vi "slow_control_2_02.vi"() -> ()   [LabVIEW 2018]
uses:
  <vilib>/DAQmx/read.llb/DAQmx Read (Analog 1D DBL NChan 1Samp).vi
  <vilib>/DAQmx/create/channels.llb/DAQmx Create Channel (AI-Voltage-Basic).vi
  <vilib>/DAQmx/miscellaneous.llb/DAQmx Fill In Error Info.vi
  <instrlib>/Lake Shore 335/Lake Shore 335.lvlib
  <instrlib>/CAEN PSM/CAEN PSM.lvlib
panel:
  out "Det.P input #":i32
  out "Flow input #":i32
  out "Coldhead":dbl
  out "Heater":dbl
  out "Cycle number":i32
  out "TOBA tester":dbl[][](array[numeric])
  in  "Cycles to execute":dbl=5.0 format="%#_13g"
  out "Moving average Det. P":dbl
  in  "N samples":i32=20
  in  "Allows tabs on \nfront panel":T1(tab)
  in  "Give name if \"Other\"":string[](array[string])
  in  "Specify input":T2(array[ring])=[enum."Detector", enum."Low", enum."High", enum."Flow", enum."None", enum."None", enum."None", enum."None"]
  in  "Multipliers":dbl[](array[numeric])=[0.2, 1.0, 1.0, 28.409091, 1.0, 1.0, 1.0, 1.0]
  in  "Offsets\nsubtracted":dbl[](array[numeric])=[0.002, 0.0, 0.0, 0.44376, 0.0, 0.0, 0.0, 0.0]
  in  "physical channels":tag[](array[tag])=["9207/ai0", "9207/ai1", "9207/ai2", "9207/ai3", "9207/ai4", "9207/ai5", "9207/ai6", "9207/ai7"]
  in  "Heater range":u16(ring) items=["Off", "Low (On)", "Medium", "High"]
  in  "Setpoint (°C)":dbl=-100.0 format="%.1f"
  in  "PID settings":cluster{"P":dbl, "I":dbl, "D":dbl}={"P"=50.0, "I"=20.0, "D"=120.0}
  in  "COM-port LakeShore":refnum<visa-resource-name>
  in  "ID Query":bool=TRUE
  in  "COM-port CAEN 1":refnum<visa-resource-name>
  in  "COM-port CAEN 2":refnum<visa-resource-name>
  out "Temp B":dbl
  out "Temp A":dbl
  out "LakeShore readings 2":dbl[](array[numeric])
  out "Converted NI9207 Readings":dbl[](array[numeric])
  in  "Run lakeshore?":bool
  out "Detector pressure":dbl
  in  "T 20":bool
  in  "T 19":bool
  in  "T 18":bool
  in  "T 17":bool
  in  "T 16":bool
  in  "T 15":bool
  in  "Detector P":bool
  in  "Overpressure threshold":dbl
  in  "Underpressure threshold":dbl
  out "Comm. status":bool
  in  "High Temp threshold":dbl format="%#_13g"
  in  "Low Temp threshold":dbl format="%#_13g"
  in  "Ignore Initialization Errors":bool=TRUE caption="Ignore init. errors?"
  out "LakeShore status":bool
  out "NI mod1 (P) status":bool
  out "CAEN 1 status":bool
  out "CAEN 2 status":bool
  out "Initialization status":bool
  out "Heater power (%)":cluster{timestamp[], dbl[]}[](graph)
  out "Flow (SLPM)":cluster{timestamp[], dbl[]}[](graph)
  out "Pressure":cluster{timestamp[], dbl[]}[](graph)
  out "Phase Diagram":cluster{"X":dbl, "Y":dbl}[](graph)
  in  "Temp. Channel selector":string(combo)="Average 15 to 20"
  out "Temperature":cluster{timestamp[], dbl[]}[](graph)
  in  "N samples":i32=30
  out "Average Flow (SLPM)":dbl caption="Average Flow (SLPM), of"
  in  "Pause?":bool
  out "Integrated Flow (SL)":dbl
  in  "Reset?":bool
  out "LakeShore readings":dbl[](array[numeric])
  out "Temp. 1":dbl
  out "Temp. 2":dbl
  out "Temp. 3":dbl
  out "Temp. 4":dbl
  out "Temp. 5":dbl
  out "Temp. 6":dbl
  out "Temp. 7":dbl
  out "Temp. 8":dbl
  out "Temp. 9":dbl
  out "Temp. 10":dbl
  out "Temp. 11":dbl
  out "Temp. 12":dbl
  out "Temp. 13":dbl
  out "Temp. 14":dbl
  out "Temp. 15":dbl
  out "Temp. 16":dbl
  out "Temp. 17":dbl
  out "Temp. 18":dbl
  out "Temp. 19":dbl
  out "Temp. 20":dbl
  out "1 to 4":dbl[](array[numeric])
  out "5 to 8":dbl[](array[numeric])
  out "9 to 12":dbl[](array[numeric])
  out "13 to 16":dbl[](array[numeric])
  out "17 to 20":dbl[](array[numeric])
  in  "Temperature Channel selector":string(combo)="Average 15 to 20"
  out "Historical Large Phase Diagram":cluster{dbl[], dbl[]}[](graph)
  out "Large Phase Diagram":cluster{"X":dbl, "Y":dbl}[](graph)
  in  "Temperature Channel selector":string(combo)="Average 15 to 20"
  in  "Set to zero":bool
  out "Bottom gate":dbl(knob) scale=0.0..-3000.0
  out "Top gate":dbl(knob) scale=0.0..3000.0
  in  "Apply Voltage":bool
  in  "VSet (V)":dbl[](array[numeric])
  in  "IMax (uA)":dbl[](array[numeric])
  in  "VMax (V)":dbl[](array[numeric])
  out "Cathode":dbl(knob) scale=0.0..-5000.0
  out "Anode":dbl(knob) scale=0.0..4000.0
  out "PMT 2":dbl(knob) scale=0.0..1000.0
  out "PMT 1":dbl(knob) scale=1.0..1000.0
  out "Vmon (V)":dbl[](array[numeric])
  out "IMon (uA)":dbl[](array[numeric])
  in  "Read V every N cycles":i16=120
  in  "Reset anode":bool
  in  "Kill every Y minutes":i32=10
  in  "Keep off for X seconds":i32=10
  out "?":bool
  out "Killed":bool
  out "Restarted":bool
  out "Anode times":dbl[](array[numeric]) format="%_12f"
  out "Anode times 2":timestamp[](array[timestamp])
  in  "Kill voltage":bool
  in  "stop":bool
  out "Voltages":dbl[](array[numeric])
  out "Started up?":bool
  out "TOBA appended":dbl[][](array[numeric])
  in  "Read T every N cycles":i32=2
  out "Time until next cycle":dbl format="%.3g"
  in  "Time per cycle (s)":i32=2 caption="Time Target (s)"
  # "<- Proof of concept for New/Old T + New P"
  # "PMT 1"
  # "PMT 2"
  # "Anode"
  # "Cathode"
  # "Top gate"
  # "Bottom gate"
  # "Connection settings"
  # "Lakeshore settings"
  # "NI 9207 Voltage settings"
  # "Gain (P) (XX.X)"
  # "Reset (I) (XX.X)"
  # "Rate (D) (X.X%)"
  # "Move to Quick Temp tab ^"
  # "Alarm indicators"
  # "Thresholds"
  # "Alarm conditions"
  # "CAEN 1"
  # "Data"
  # "PMT 1"
  # "PMT 1"
  # "PMT 2"
  # "PMT 2"
  # "Anode"
  # "Anode"
  # "Cathode"
  # "Cathode"
  # "Top gate"
  # "Top gate"
  # "Bottom gate"
  # "Bottom gate"
  # "Settings"
  # "PMT 1"
  # "PMT 1"
  # "PMT 2"
  # "PMT 2"
  # "Anode"
  # "Anode"
  # "Cathode"
  # "Cathode"
  # "Top gate"
  # "Top gate"
  # "Bottom gate"
  # "Bottom gate"
  # "CAEN 2"
  # "PMT 1"
  # "PMT 2"
  # "Anode"
  # "Cathode"
  # "Needle gauges or other displays go here"
  # "Top gate"
  # "Bottom gate"
  # "Time of last reset"
  # "Time of last reactivation"
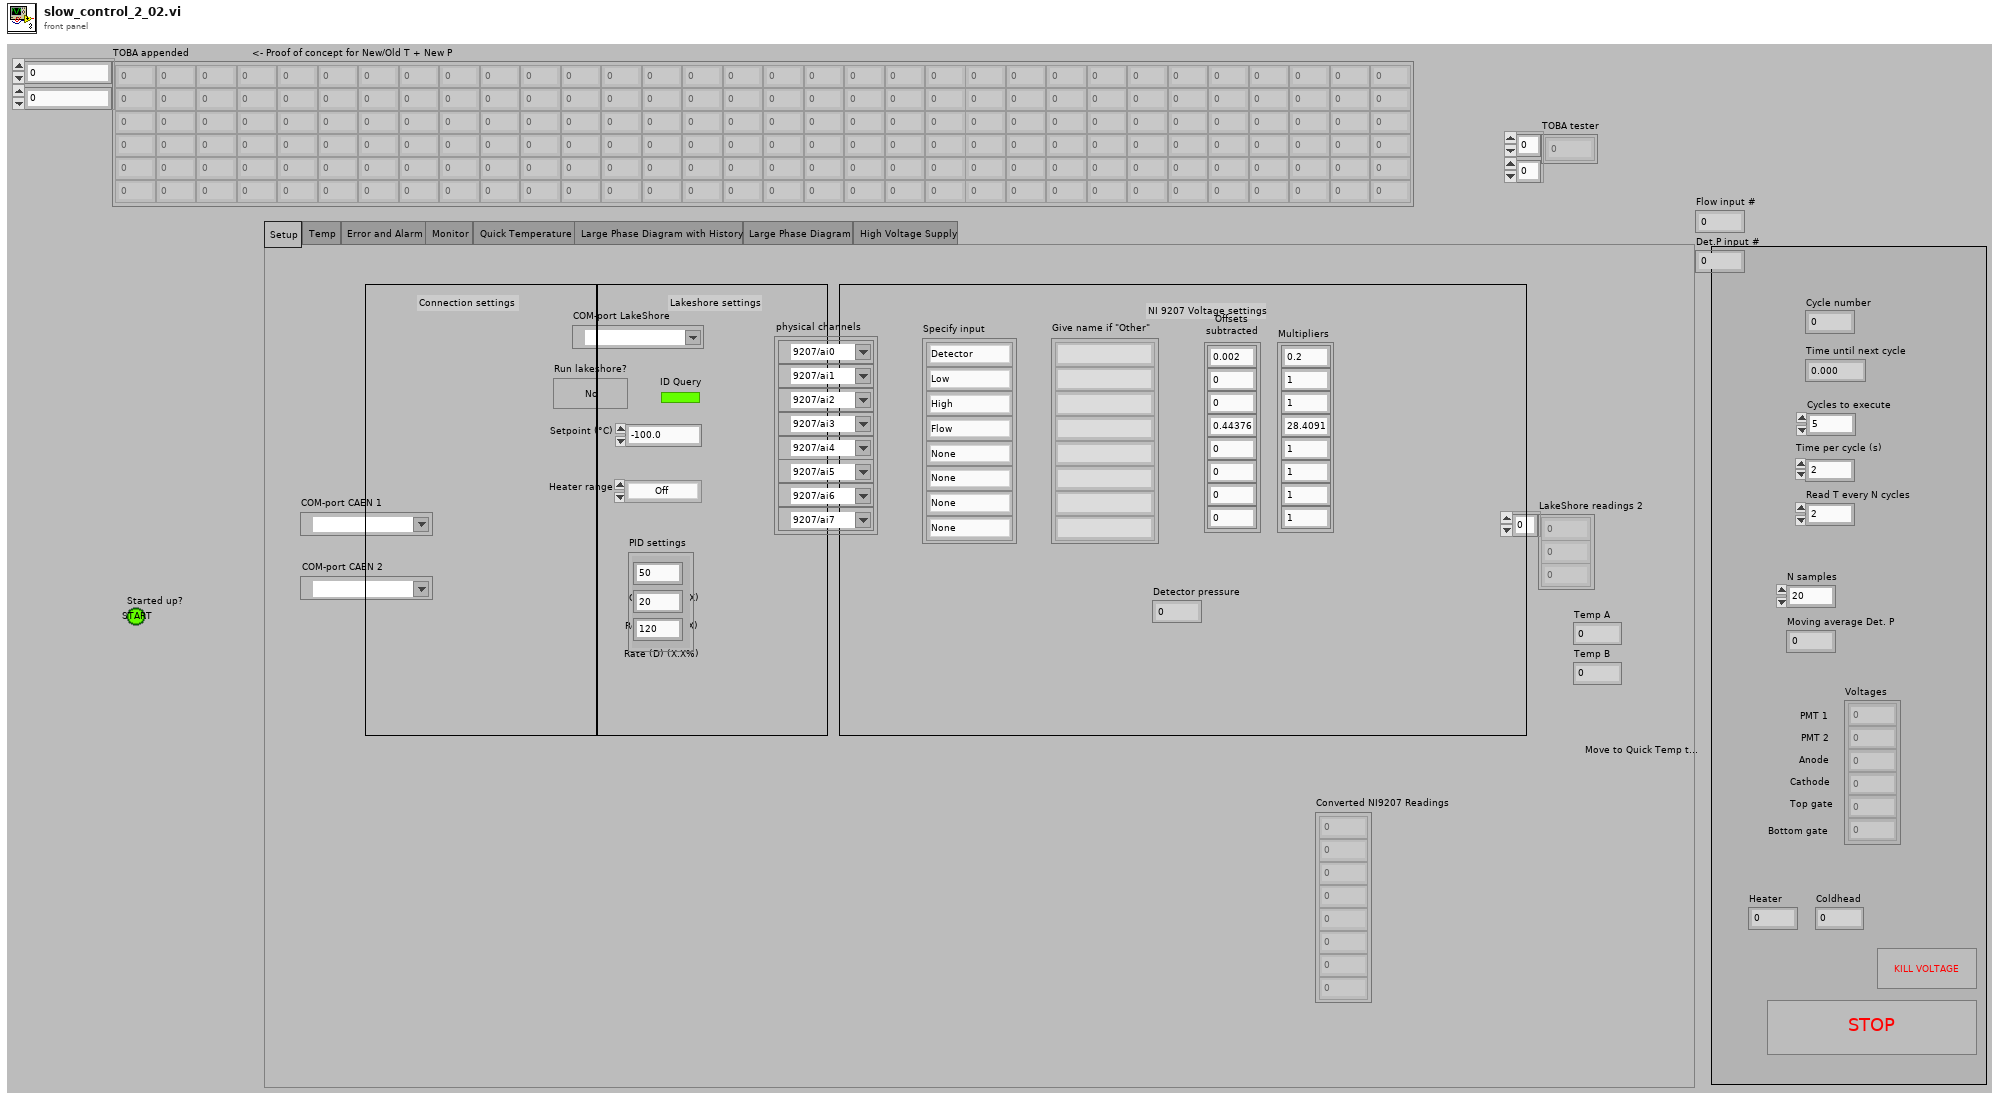
[diagram p1: front panel]
types:
  T1 = enum32{"Setup", "Temp", "Error and Alarm", "Monitor", "Quick Temperature", "Large Phase Diagram with History", "Large Phase Diagram", "High Voltage Supply"}
  T2 = enum16{"Detector", "Low", "High", "Flow", "Other", "None"}[]
  T3 = enum16{"Detector", "Low", "High", "Flow", "Other", "None"}
  T4 = cluster{"Baud Rate":u32, "Parity":u16, "Data Bits":u16, "Stop Bits":u16, "Flow Control":u16}
  T5 = cluster{"VISA resource name out":refnum<visa-resource-name>, "error out":errorcluster}
  T6 = cluster{"task out":refnum<k21>, "error out":errorcluster}
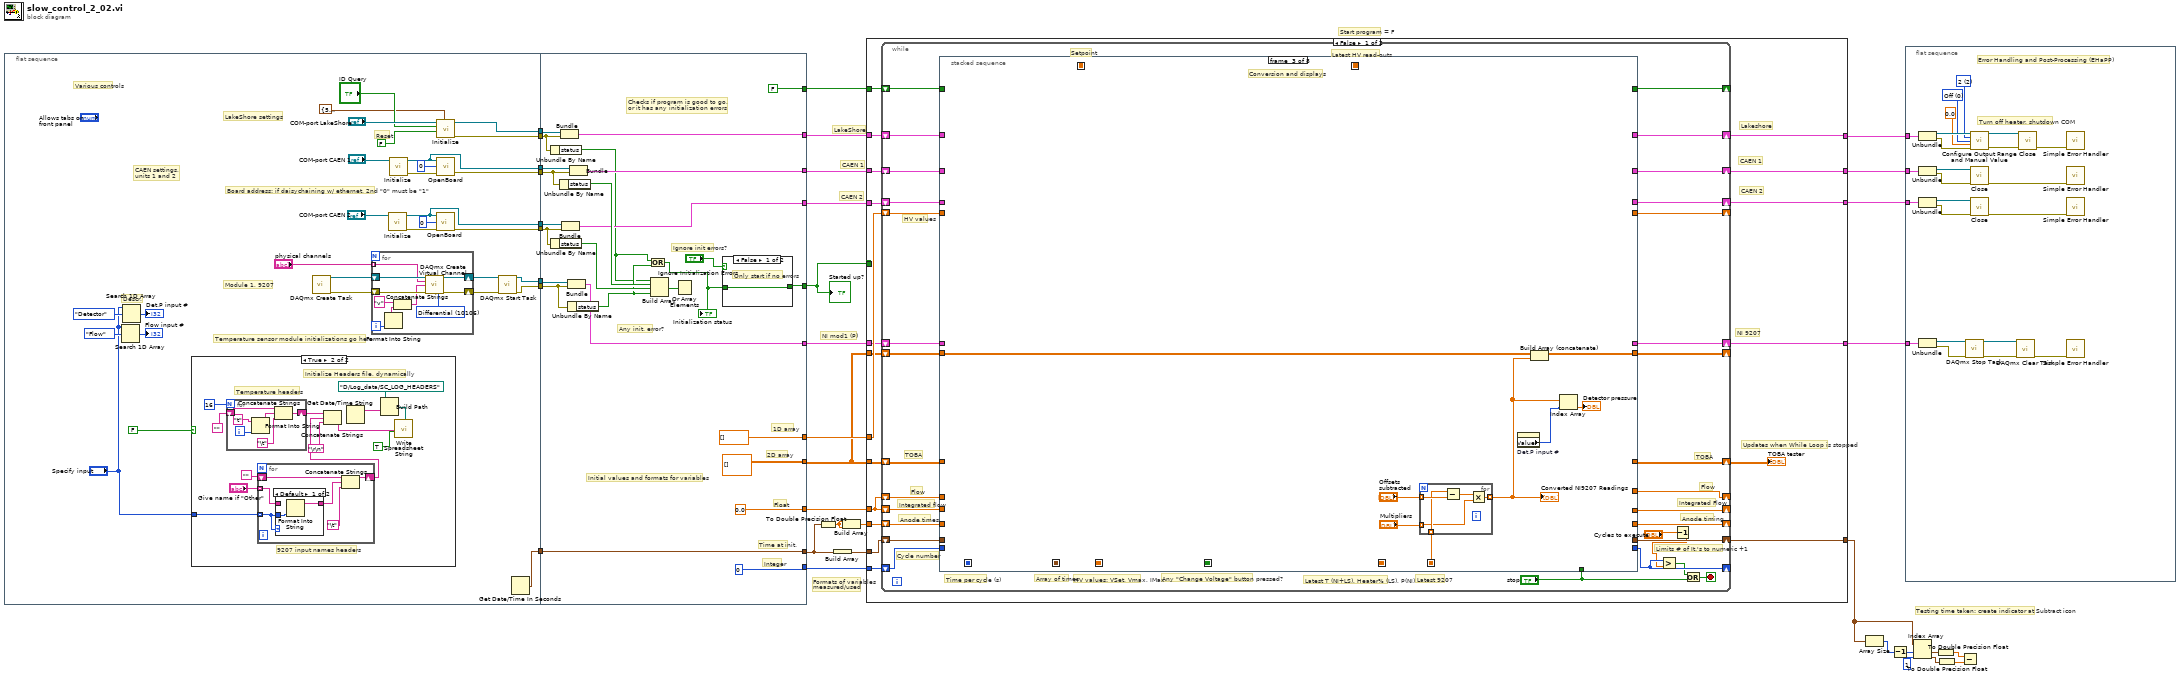
[diagram p0: block diagram]
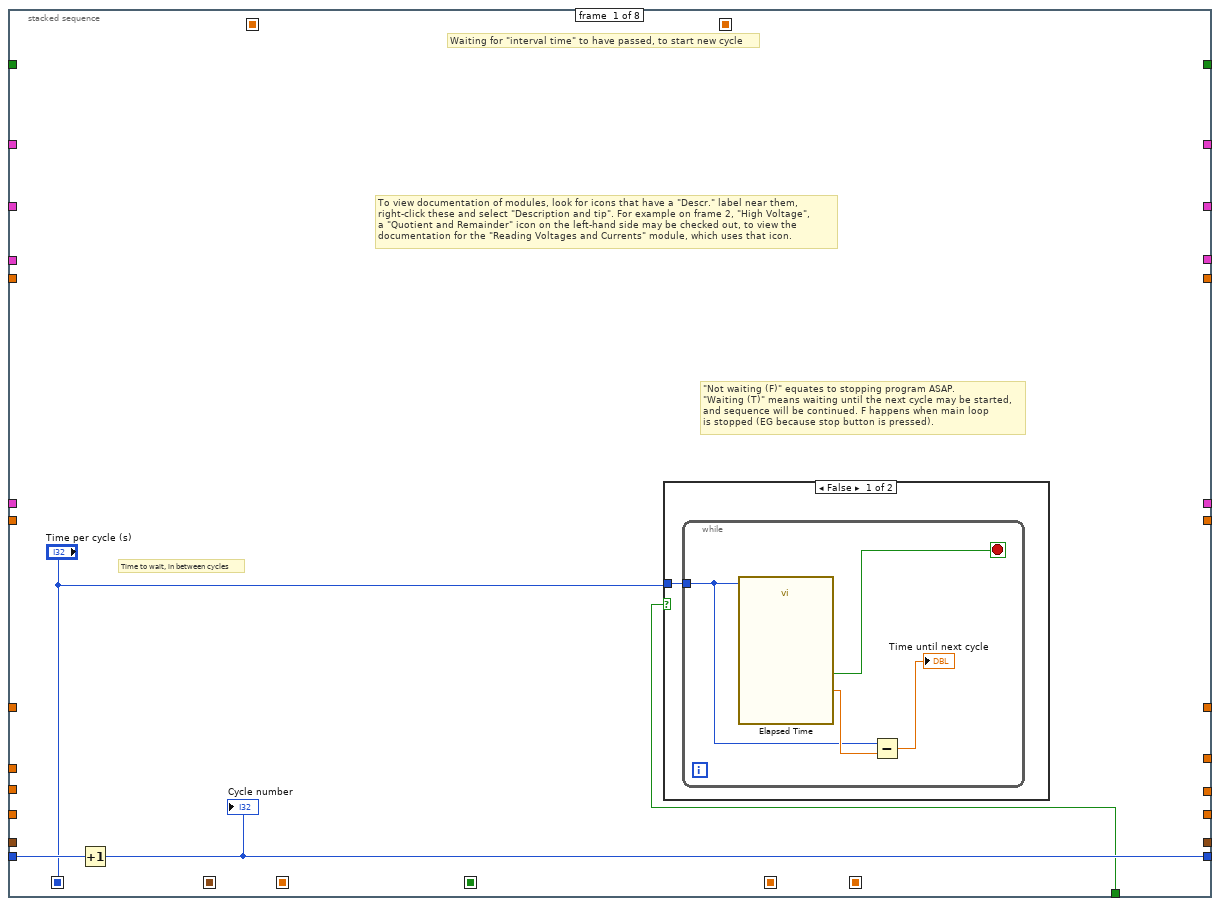
[diagram p2: hidden frame]
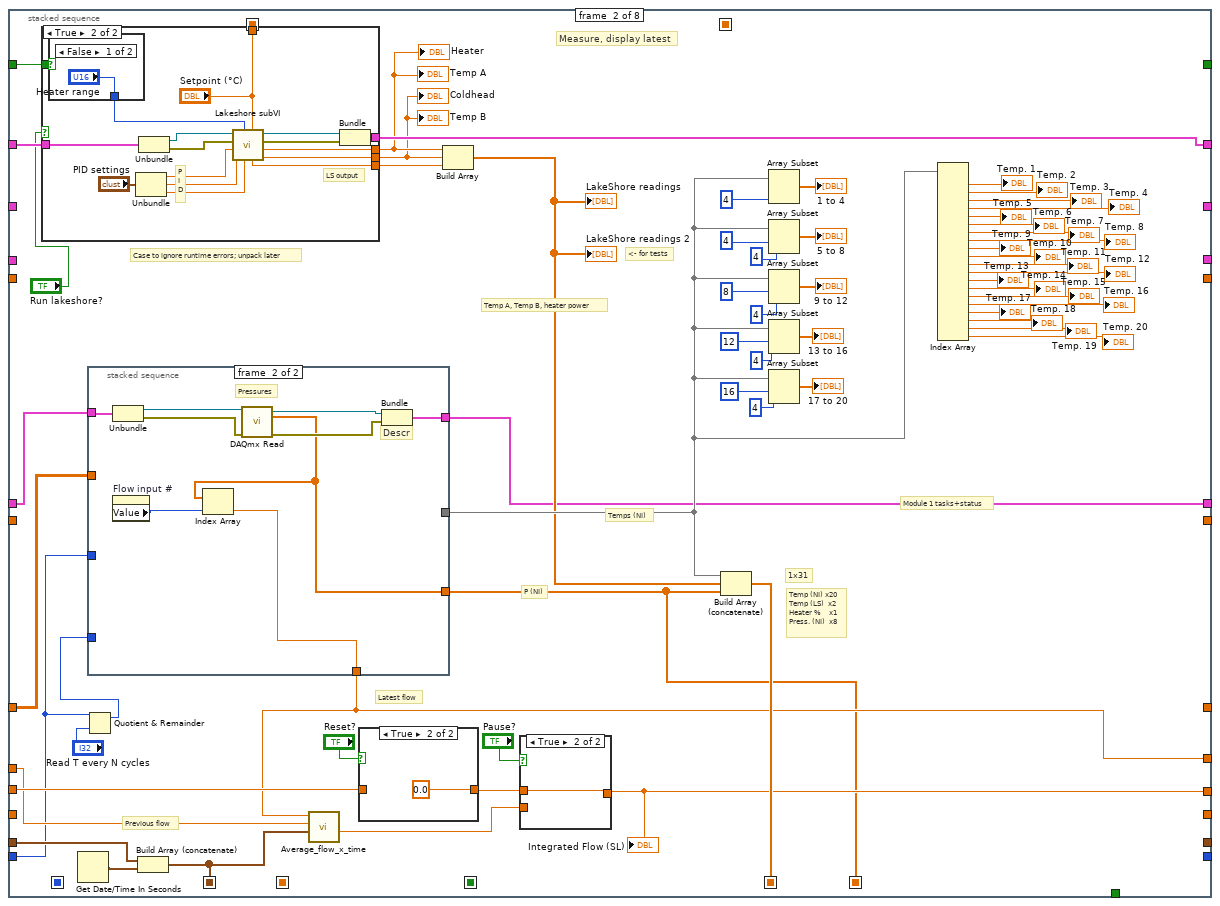
[diagram p4: hidden frame]
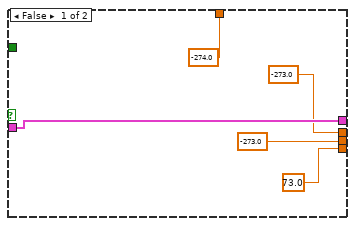
[diagram p5: hidden frame]
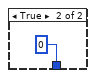
[diagram p6: hidden frame]
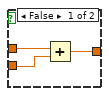
[diagram p8: hidden frame]
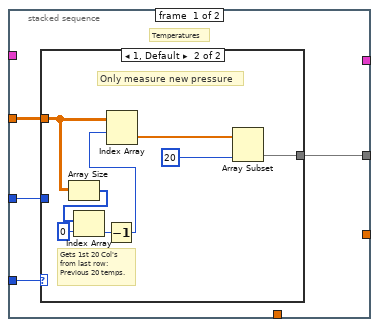
[diagram p9: hidden frame]
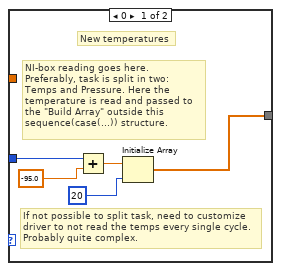
[diagram p10: hidden frame]
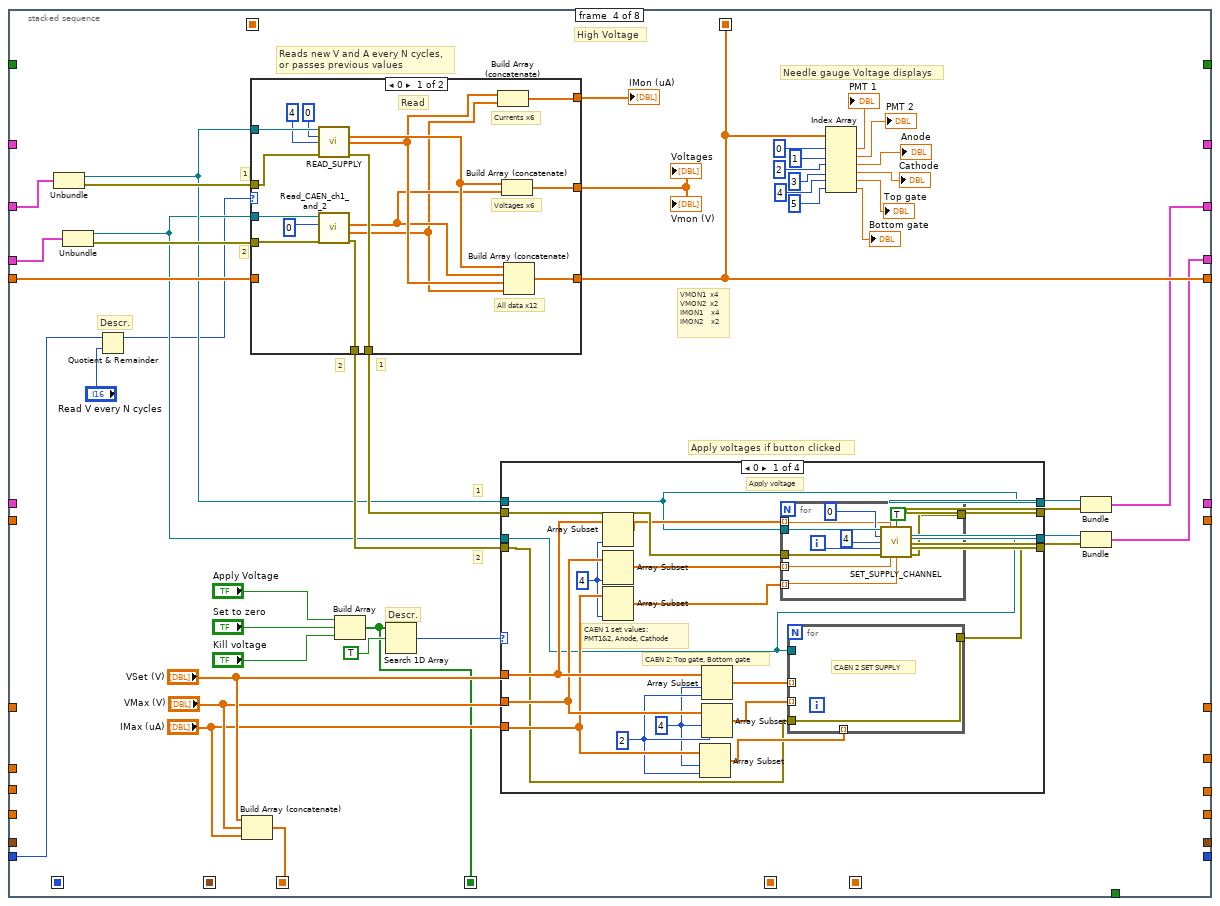
[diagram p11: hidden frame]
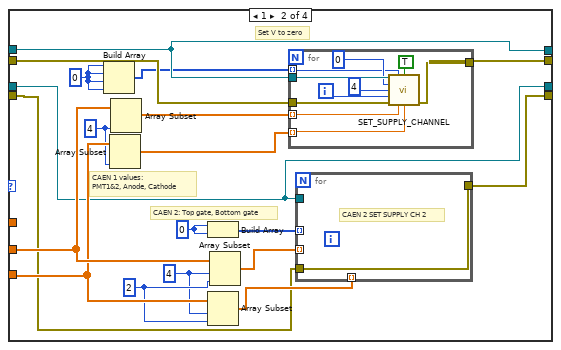
[diagram p12: hidden frame]
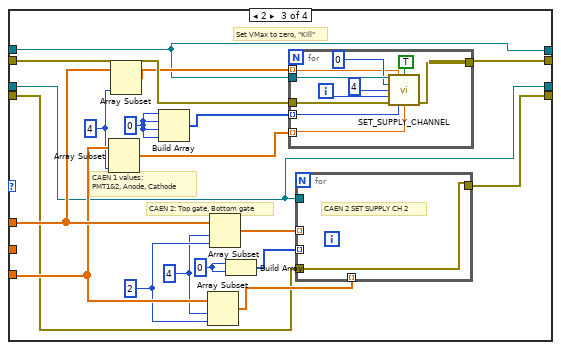
[diagram p13: hidden frame]
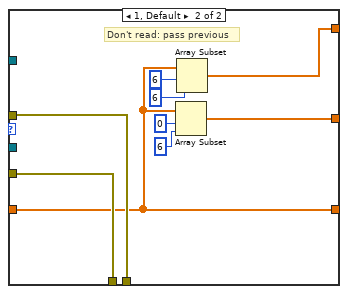
[diagram p15: hidden frame]
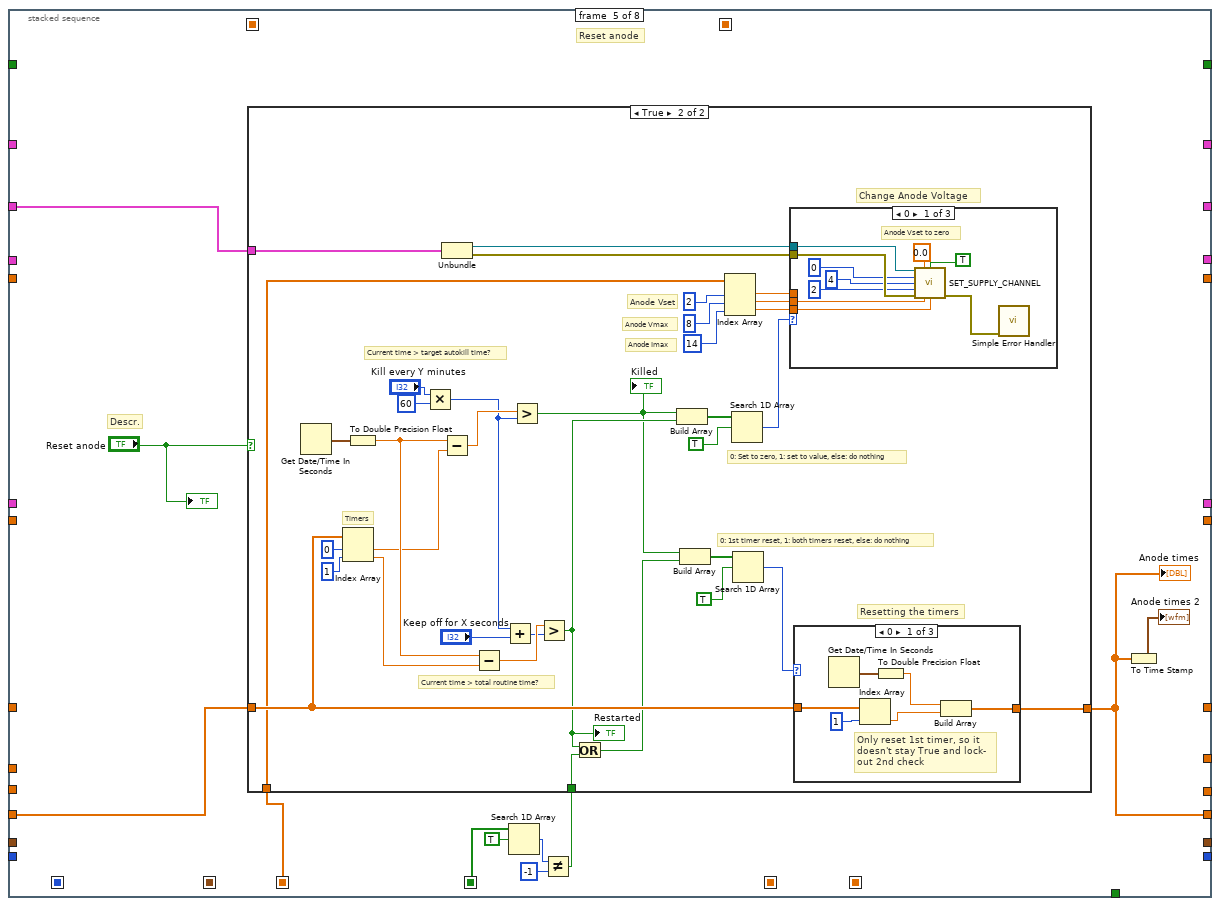
[diagram p16: hidden frame]
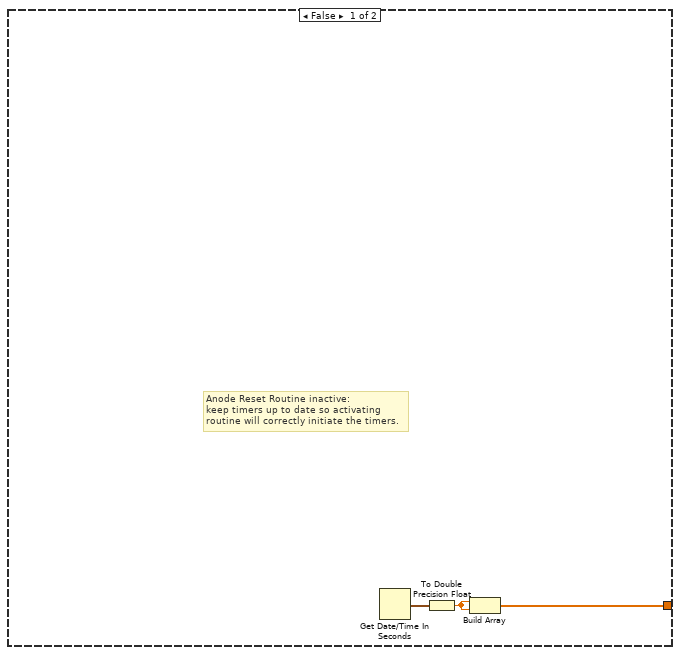
[diagram p17: hidden frame]
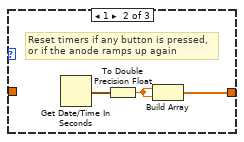
[diagram p18: hidden frame]
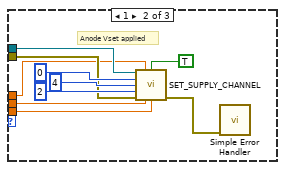
[diagram p20: hidden frame]
diagram:
  # "Testing time taken: create indicator at Subtract icon"
  # "NI mod1 (P)"
  # "Start program = F"
  # "CAEN 2"
  # "CAEN 1"
  # "LakeShore"
  # "Formats of variables\nmeasured/used"
  n1 = flat-sequence {
    tunnel: [w62] -> w35
    tunnel: [w61] -> w34
    tunnel: [w48] -> w33
    tunnel: [w58] -> w32
    tunnel: [w37] -> w31
    tunnel: [w57] -> w26
    tunnel: [w53] -> w18
    tunnel: [w52] -> w17
    tunnel: [w38] -> w8
    tunnel: w35 -> [w126]
    tunnel: w34 -> [w125]
    tunnel: w33 -> [w123]
    tunnel: w32 -> [w122]
    tunnel: w31 -> [w112]
    tunnel: [w127] -> w15
    tunnel: [0.0] -> w14
    tunnel: [dbl[] []] -> w30
    tunnel: [dbl[][] []] -> w1
    tunnel: [0] -> w29
    tunnel: [w124] -> w28
    tunnel: [w121] -> w27
    tunnel: [w120] -> w13
    tunnel: w26 -> [w120]
    tunnel: w18 -> [w118]
    tunnel: w17 -> [w117]
    tunnel: [w116] -> w16
    tunnel: [FALSE] -> w9
    tunnel: w8 -> [w113]
    tunnel: [w111] -> w7
    frame #0 {
      # "Descr."
      # "Various controls"
      # "Temperature sensor module initializations go here"
      # "Module 1, 9207"
      # "Board address: if daisychaining w/ ethernet, 2nd \"0\" must be \"1\""
      # "CAEN settings,\nunits 1 and 2"
      # "Reset"
      # "LakeShore settings"
      n2 = Search 1D Array(1D array="Specify input", element=T3."Flow") -> (index of element=→"Flow input #":i32)  [unwired: 1 in]
      n3 = Search 1D Array(1D array="Specify input", element=T3."Detector") -> (index of element=→"Det.P input #":i32)  [unwired: 1 in]
      n4 = case shown="True" FALSE {
        tunnel: "Specify input" -> [_ w84]
        frame False {
        }
        frame True {
          # "9207 input names headers"
          # "Temperature headers"
          # "Initialize Headers file, dynamically"
          n5 = for {
            N: 16 -> [_]
            shift-right: [w98] -> w79
            shift-left: "" -> [w99]
            i -> [w103]
            n6 = Format Into String(initial string="t", w103) -> (resulting string=w101:string)  [unwired: 2 in, 1 out]
            n7 = Concatenate Strings(w99, w101, "\t") -> (w98:string)
          }
          n8 = for {
            tunnel: w84 -> [w90] mode=indexing
            shift-right: [w91] -> w76
            shift-left: "" -> [w92]
            tunnel: "Give name if \"Other\"" -> [w94] mode=indexing
            n9 = case shown="Default" w90 {
              tunnel: w94 -> [_ w97]
              tunnel: [w95 w97] -> w93
              tunnel: w90 -> [w96 _]
              frame Default {
                n10 = Format Into String(w96) -> (resulting string=w95:string)  [unwired: 3 in, 1 out]
              }
              frame "Other" {
              }
            }
            n11 = Concatenate Strings(w92, w93, "\t") -> (w91:string)
          }
          n12 = Concatenate Strings(w79, w76, "\r\n") -> (w77:string)
          n13 = Get Date/Time String() -> (date string=w82:string)  [unwired: 3 in, 1 out]
          n14 = Build Path(base path=path "D:/Log_data/SC_LOG_HEADERS" ("file path (dialog if empty)"), name or relative path=w82) -> (appended path=w83:path)
          n15 = call <vilib>:"Write Spreadsheet String.vi"("append to file? (new file:F)"=TRUE, "spreadsheet string"=w77, "file path (dialog if empty)"=w83) -> ()  [unwired: 7 in, 2 out]
        }
      }
      n16 = call <vilib>:"DAQmx Create Task.vi"() -> ("task out"=w47:refnum<k21>, "error out"=w46:errorcluster)  [unwired: 14 in]
      n17 = for {
        shift-right: [w71] -> w40
        shift-left: w47 -> [w70]
        shift-right: [w72] -> w39
        shift-left: w46 -> [w68]
        tunnel: "physical channels" -> [w69] mode=indexing
        i -> [w74]
        w66 = 10106 items=["Default"=-1, "RSE"=10083, "NRSE"=10078, "Differential"=10106, "Pseudodifferential"=12529] ("input terminal configuration")
        n18 = Format Into String(w74) -> (resulting string=w73:string)  [unwired: 3 in, 1 out]
        n19 = Concatenate Strings("v" ("string"), w73) -> (w67:string)
        n20 = call-poly <vilib>:"DAQmx Create Virtual Channel.vi"("task in"=w70, "input terminal configuration"=w66, "physical channels"=w69, "name to assign"=w67, "error in"=w68) -> ("task out"=w71:refnum<k21>, "error out"=w72:errorcluster)  [unwired: 9 in]
      }
      n21 = call <instrlib>:"Initialize.vi"("VISA resource name"="COM-port CAEN 2") -> ("error out"=w54:errorcluster, "VISA resource name out"=w53:refnum<visa-resource-name>)  [unwired: 9 in]
      n22 = call <instrlib>:"Initialize.vi"("VISA resource name"="COM-port CAEN 1") -> ("error out"=w59:errorcluster, "VISA resource name out"=w48:refnum<visa-resource-name>)  [unwired: 9 in]
      n23 = call <instrlib>:"OpenBoard.vi"("error in (no error)"=w54, "Board Address"=u8 0, "VISA resource name"=w53) -> ("error out"=w52:errorcluster)  [unwired: 7 in, 1 out]
      n24 = call <instrlib>:"Initialize.vi"("Serial Configuration"=T4 {"Baud Rate"=57600, "Parity"=1, "Data Bits"=7, "Stop Bits"=10, "Flow Control"=0}, "Reset (True)"=FALSE ("Reset (LakeShore)"), "ID Query (True)"="ID Query", "VISA resource name"="COM-port LakeShore") -> ("error out"=w61:errorcluster, "VISA resource name out"=w62:refnum<visa-resource-name>)  [unwired: 6 in]
      n25 = call <instrlib>:"OpenBoard.vi"("error in (no error)"=w59, "Board Address"=0, "VISA resource name"=w48) -> ("error out"=w58:errorcluster)  [unwired: 7 in, 1 out]
      n26 = call <vilib>:"DAQmx Start Task.vi"("task/channels in"=w40, "error in"=w39) -> ("task out"=w38:refnum<k21>, "error out"=w37:errorcluster)  [unwired: 12 in]
      n27 = Get Date/Time In Seconds() -> (seconds since 1Jan1904=w57:timestamp)
    }
    frame #1 {
      # "Initial values and formats for variables"
      # "Time at init."
      # "Integer"
      # "2D array"
      # "1D array"
      # "Float"
      # "Checks if program is good to go,\nor it has any initialization errors"
      # "Ignore init errors?"
      # "Any init. error?"
      n28 = Unbundle By Name(w125) -> ("status"=w105:bool)
      n29 = Unbundle By Name(w117) -> ("status"=w119:bool)
      n30 = Unbundle By Name(w122) -> ("status"=w128:bool)
      n31 = Bundle("VISA resource name out"=w126, "error out"=w125) -> (w124:T5)  [unwired: 1 in]
      n32 = Bundle("VISA resource name out"=w118, "error out"=w117) -> (w116:T5)  [unwired: 1 in]
      n33 = Unbundle By Name(w112) -> ("status"=w106:bool)
      n34 = Bundle("task out"=w113, "error out"=w112) -> (w111:T6)  [unwired: 1 in]
      n35 = Bundle("VISA resource name out"=w123, "error out"=w122) -> (w121:T5)  [unwired: 1 in]
      n36 = Or(x=w105, y=w106) -> (x .or. y?=w104:bool)
      "Initialization status" <- w104
      n37 = Build Array(w105, w128, w106, w119) -> (w129:bool[])
      n38 = Or Array Elements(Boolean array=w129) -> ()  [unwired: 1 out]
      n39 = case shown="False" "Ignore Initialization Errors" {
        tunnel: [w130 FALSE] -> w127
        tunnel: w104 -> [w130 _]
        frame False {
          # "Only start if no errors"
        }
        frame True {
          # "Always start program"
        }
      }
    }
  }
  n40 = To Double Precision Float(number=w13) -> (double precision float=w12:dbl)
  n41 = Build Array(w13) -> (w25:timestamp[])
  n42 = Build Array(w12, w12) -> (w11:dbl[])
  n43 = case shown="False" w15 {
    selector: w15 -> [_ w759]
    tunnel: [_ w759] -> _
    tunnel: w30 -> [w142 _]
    tunnel: w29 -> [w149 _]
    tunnel: w1 -> [w148 _]
    tunnel: w28 -> [w143 w757]
    tunnel: w27 -> [w145 w756]
    tunnel: w25 -> [w147 _]
    tunnel: [w146 timestamp[] []] -> w21
    tunnel: w16 -> [w144 w755]
    tunnel: w14 -> [w137 _]
    tunnel: w11 -> [w141 _]
    tunnel: [w139 w757] -> w10
    tunnel: w9 -> [w138 _]
    tunnel: w7 -> [w136 w754]
    tunnel: [w135 w756] -> w6
    tunnel: [w134 w755] -> w5
    tunnel: [w133 w754] -> w4
    tunnel: w1 -> [w132 _]
    frame False {
      # "NI 9207"
      # "CAEN 2"
      # "CAEN 1"
      # "Lakeshore"
      # "Updates when While Loop is stopped"
      n44 = while {
        shift-right: [w175] -> _
        shift-left: w149 -> [w180]
        shift-right: [w177] -> w140
        shift-left: w148 -> [w166]
        shift-right: [w167] -> w146
        shift-left: w147 -> [w176]
        shift-right: [w169] -> w135
        shift-left: w145 -> [w158]
        shift-right: [w171] -> _
        shift-left: w142 -> [w174]
        shift-right: [w168] -> w134
        shift-left: w144 -> [w173]
        shift-right: [w170] -> w139
        shift-left: w143 -> [w172]
        shift-right: [w165] -> _
        shift-left: w137 -> [w160]
        shift-right: [w162] -> _
        shift-left: w137 -> [w161]
        shift-right: [w157] -> _
        shift-left: w141 -> [w159]
        shift-right: [w155] -> _
        shift-left: w138 -> [w156]
        shift-right: [w153] -> w133
        shift-left: w136 -> [w154]
        shift-right: [w151] -> _
        shift-left: w132 -> [w152]
        stop <- w178 stop-if-true
        # "Latest 9207"
        # "Any \"Change Voltage\" button pressed?"
        # "Setpoint"
        # "Anode timing"
        # "Anode times"
        # "Integrated flow"
        # "Flow"
        # "Flow"
        # "Integrated Flow"
        # "TOBA"
        # "Array of times"
        # "Latest HV read-outs"
        # "Time per cycle (s)"
        # "Cycle number"
        # "HV values: VSet, Vmax, IMax"
        # "HV values"
        # "TOBA"
        # "Latest T (NI+LS), Heater% (LS), P(NI)"
        # "Limits # of It.'s to numeric +1"
        n45 = stacked-sequence {
          seq-local: [_ w250 _ _ _ _ _ _] -> [_ _ _ _ _ w597 w715 w727]
          seq-local: [_ _ _ w327 _ _ _ _] -> [_ _ _ _ w489 _ _ _]
          seq-local: ["Time per cycle (s)" _ _ _ _ _ _ _] -> [_ _ _ _ _ _ w711 _]
          seq-local: [_ _ _ w342 _ _ _ _] -> [_ _ _ _ _ _ w710 _]
          seq-local: [_ w206 _ _ _ _ _ _] -> [_ _ _ _ _ w577 _ _]
          seq-local: [_ _ _ w321 _ _ _ _] -> [_ _ _ _ w492 _ _ _]
          seq-local: [_ w191 _ _ _ _ _ _] -> [_ _ _ _ _ _ w714 _]
          seq-local: [_ w193 _ _ _ _ _ _] -> [_ _ w314 _ _ _ _ _]
          tunnel: [w183 _ _ _ _ _ _ _] -> w175
          tunnel: "stop" -> [w182 _ _ _ _ _ _ _]
          tunnel: w180 -> [w184 w195 _ w356 _ _ _ _]
          tunnel: w166 -> [_ w251 _ _ _ w604 _ _]
          tunnel: [_ _ _ _ _ w562 _ _] -> w177
          tunnel: w176 -> [_ w247 _ _ _ _ _ _]
          tunnel: w158 -> [_ _ _ w363 w490 _ _ w746]
          tunnel: w174 -> [_ _ _ w361 _ _ _ _]
          tunnel: w173 -> [_ _ _ w360 _ _ _ w745]
          tunnel: w172 -> [_ w248 _ _ _ _ _ w744]
          tunnel: [_ w249 _ _ _ _ _ _] -> w170
          tunnel: [_ _ _ w342 _ _ _ _] -> w171
          tunnel: [_ _ _ w335 _ _ _ _] -> w169
          tunnel: [_ _ _ w332 _ _ _ _] -> w168
          tunnel: [_ _ _ _ _ w577 _ _] -> w167
          tunnel: w160 -> [_ w242 _ _ _ _ _ _]
          tunnel: [_ w243 _ _ _ _ _ _] -> w165
          tunnel: [_ w204 _ _ _ _ _ _] -> w162
          tunnel: w161 -> [_ w203 _ _ _ _ _ _]
          tunnel: w159 -> [_ _ _ _ w491 _ _ _]
          tunnel: [_ _ _ _ w485 _ _ _] -> w157
          tunnel: w156 -> [_ w198 _ _ _ _ _ _]
          tunnel: [_ _ _ _ _ _ _ FALSE] -> w155
          tunnel: w154 -> [_ w197 _ _ _ _ _ w742]
          tunnel: [_ w196 _ _ _ _ _ _] -> w153
          tunnel: w152 -> [_ _ w312 _ _ _ _ _]
          tunnel: [_ _ w311 _ _ _ _ _] -> w151
          frame #0 {
            # "To view documentation of modules, look for icons that have a \"Descr.\" label near them,\nright-click these and select \"Description and tip\". For example on frame 2, \"High Voltage\",\na \"Quotient and Remainder\" icon on the left-hand side may be checked out, to view the\ndocumentation for the \"Reading Voltages and Currents\" module, which uses that icon."
            # "Time to wait, in between cycles"
            # "\"Not waiting (F)\" equates to stopping program ASAP.\n\"Waiting (T)\" means waiting until the next cycle may be started,\nand sequence will be continued. F happens when main loop \nis stopped (EG because stop button is pressed)."
            # "Waiting for \"interval time\" to have passed, to start new cycle"
            n46 = Increment(x=w184) -> (x+1=w183:i32)
            "Cycle number" <- w183
            n47 = case shown="False" w182 {
              tunnel: "Time per cycle (s)" -> [w185 _]
              frame False {
                n48 = while {
                  tunnel: w185 -> [w187]
                  stop <- w189 stop-if-true
                  n49 = call "Elapsed Time"("Time Target (s)"=w187) -> ("Elapsed Time (s)"=w188:dbl, "Time has Elapsed"=w189:bool)  [unwired: 11 in, 6 out]
                  n50 = Subtract(x=w187, y=w188) -> (x-y=→"Time until next cycle":dbl)
                }
              }
              frame True {
              }
            }
          }
          frame #1 {
            # "Case to ignore runtime errors; unpack later"
            # "Previous flow"
            # "Latest flow"
            # "Module 1 tasks+status"
            # "<- for tests"
            # "P (NI)"
            # "Temps (NI)"
            # "1x31"
            # "Temp (NI) x20\nTemp (LS)  x2\nHeater %    x1\nPress. (NI)  x8"
            # "Temp A, Temp B, heater power"
            # "Measure, display latest"
            n51 = case shown="True" "Run lakeshore?" {
              tunnel: [w256 w264] -> w249
              tunnel: w248 -> [w256 w263]
              tunnel: [-273.0 ("Input A") w262] -> w202
              tunnel: [-273.0 ("Input B") w261] -> w201
              tunnel: [73.0 ("Heater 1 (%)") w260] -> w200
              tunnel: w198 -> [_ w259]
              tunnel: [-274.0 "Setpoint (°C)"] -> w191
              frame False {
              }
              frame True {
                # "LS output"
                # "P\nI\nD"
                n52 = case shown="False" w259 {
                  tunnel: ["Heater range" 0] -> w267
                  frame False {
                  }
                  frame True {
                  }
                }
                n53 = Unbundle("PID settings") -> ("P"=w270:dbl, "I"=w269:dbl, "D"=w268:dbl)
                n54 = Unbundle(w263) -> ("VISA resource name out"=w272:refnum<visa-resource-name>, "error out"=w271:errorcluster)
                n55 = call "Lakeshore subVI.vi"("Setpoint"="Setpoint (°C)", "Rate (D) (X.X %)"=w268, "Range"=w267, "Reset (I) (XX.X)"=w269, "Gain (P) (XX.X)"=w270, "error in (no error)"=w271, "VISA resource name"=w272) -> ("Input B"=w261:dbl, "Input A"=w262:dbl, "error out"=w265:errorcluster, "VISA resource name out"=w266:refnum<visa-resource-name>, "Heater 1 (%)"=w260:dbl)
                n56 = Bundle("VISA resource name out"=w266, "error out"=w265) -> (w264:T5)  [unwired: 1 in]
              }
            }
            "Temp A" <- w202
            "Temp B" <- w201
            "Coldhead" <- w201
            "Heater" <- w202
            n57 = Get Date/Time In Seconds() -> (seconds since 1Jan1904=w246:timestamp)
            n58 = Quotient & Remainder(x=w195, y="Read T every N cycles") -> (x-y*floor(x/y)=w190:i32)  [unwired: 1 out]
            n59 = stacked-sequence {
              tunnel: w190 -> [w285 _]
              tunnel: [w284 _] -> w205
              tunnel: [_ w301] -> w193
              tunnel: w251 -> [w283 _]
              tunnel: w195 -> [w282 _]
              tunnel: [_ w300] -> w204
              tunnel: w197 -> [_ w307]
              tunnel: [_ w302] -> w196
              frame #0 {
                # "Temperatures"
                n60 = case shown="1, Default" w285 {
                  tunnel: w283 -> [_ w295]
                  tunnel: [w288 w291] -> w284
                  tunnel: w282 -> [w287 _]
                  frame 0 {
                    # "If not possible to split task, need to customize\ndriver to not read the temps every single cycle.\nProbably quite complex."
                    # "NI-box reading goes here.\nPreferably, task is split in two: \nTemps and Pressure. Here the \ntemperature is read and passed to \nthe \"Build Array\" outside this \nsequence(case(...)) structure."
                    # "New temperatures"
                    n61 = Add(x=w287, y=-95.0 ("element")) -> (x+y=w290:dbl)
                    n62 = Initialize Array(w290, 20) -> (w288:dbl[])
                  }
                  frame 1, Default {
                    # "Gets 1st 20 Col's\nfrom last row:\nPrevious 20 temps."
                    # "Only measure new pressure"
                    n63 = Array Size(array=w295) -> (size(s)=w297:i32[])
                    n64 = Index Array(array=w297, index=0) -> (element=w298:i32)
                    n65 = Decrement(x=w298) -> (x-1=w294:i32)
                    n66 = Index Array(array=w295, index (row)=w294) -> (element=w293:dbl[])  [unwired: 1 in]
                    n67 = Array Subset(array=w293, length=20) -> (w291:dbl[])  [unwired: 1 in]
                  }
                }
              }
              frame #1 {
                # "Descr"
                # "Pressures"
                n68 = Unbundle(w307) -> ("task out"=w306:refnum<k21>, "error out"=w305:errorcluster)
                n69 = property on="Flow input #" class="DigNum (strict)"() -> ("Value"=w299:i32)  [unwired: 2 in, 2 out]
                n70 = call-poly <vilib>:"DAQmx Read.vi"("task/channels in"=w306, "error in"=w305) -> ("task out"=w304:refnum<k21>, "data"=w301:dbl[], "error out"=w303:errorcluster)  [unwired: 11 in]
                n71 = Index Array(array=w301, index=w299) -> (element=w300:dbl)
                n72 = Bundle("task out"=w304, "error out"=w303) -> (w302:T6)  [unwired: 1 in]
              }
            }
            n73 = Build Array (concatenate)(w247, w246) -> (w206:timestamp[])
            n74 = call "Average_flow_x_time.vi"("Array of timestamps"=w206, "Previous Flow"=w203, "Latest Flow"=w204) -> ("Volume (SL)"=w194:dbl)  [unwired: 8 in]
            n75 = case shown="True" "Reset?" {
              tunnel: w242 -> [w276 _]
              tunnel: [w276 0.0] -> w241
              frame False {
              }
              frame True {
              }
            }
            n76 = Build Array(w202, w201, w200) -> (w199:dbl[])
            "LakeShore readings" <- w199
            "LakeShore readings 2" <- w199
            n77 = case shown="True" "Pause?" {
              tunnel: w194 -> [w280 _]
              tunnel: w241 -> [w279 w281]
              tunnel: [w278 w281] -> w243
              frame False {
                n78 = Add(x=w279, y=w280) -> (x+y=w278:dbl)
              }
              frame True {
              }
            }
            "Integrated Flow (SL)" <- w243
            n79 = Build Array (concatenate)(w205, w199, w193) -> (w250:dbl[])
            n80 = Array Subset(array=w205, length=4) -> (→"1 to 4":dbl[])  [unwired: 1 in]
            n81 = Array Subset(array=w205, index=4, length=4 ("index")) -> (→"5 to 8":dbl[])
            n82 = Array Subset(array=w205, index=8, length=4 ("index")) -> (→"9 to 12":dbl[])
            n83 = Array Subset(array=w205, index=12, length=4 ("index")) -> (→"13 to 16":dbl[])
            n84 = Array Subset(array=w205, index=16, length=4 ("index")) -> (→"17 to 20":dbl[])
            n85 = Index Array(array=w205) -> (element #1=→"Temp. 1":dbl, element #2=→"Temp. 2":dbl, element #3=→"Temp. 3":dbl, element #4=→"Temp. 4":dbl, element #5=→"Temp. 5":dbl, element #6=→"Temp. 6":dbl, element #7=→"Temp. 7":dbl, element #8=→"Temp. 8":dbl, element #9=→"Temp. 9":dbl, element #10=→"Temp. 10":dbl, element #11=→"Temp. 11":dbl, element #12=→"Temp. 12":dbl, element #13=→"Temp. 13":dbl, element #14=→"Temp. 14":dbl, element #15=→"Temp. 15":dbl, element #16=→"Temp. 16":dbl, element #17=→"Temp. 17":dbl, element #18=→"Temp. 18":dbl, element #19=→"Temp. 19":dbl, element #20=→"Temp. 20":dbl)  [unwired: 20 in]
          }
          frame #2 {
            # "Conversion and displays"
            n86 = for {
              tunnel: "Offsets\nsubtracted" -> [w320] mode=indexing
              tunnel: w314 -> [w319] mode=indexing
              tunnel: "Multipliers" -> [w317] mode=indexing
              tunnel: [w316] -> w310 mode=indexing
              n87 = Subtract(x=w319, y=w320) -> (x-y=w318:dbl)
              n88 = Multiply(x=w318, y=w317) -> (x*y=w316:dbl)
            }
            "Converted NI9207 Readings" <- w310
            n89 = property on="Det.P input #" class="DigNum (strict)"() -> ("Value"=w308:i32)  [unwired: 2 in, 2 out]
            n90 = Build Array (concatenate)(w312, w310) -> (w311:dbl[][])
            n91 = Index Array(array=w310, index=w308) -> (element=→"Detector pressure":dbl)
          }
          frame #3 {
            # "Apply voltages if button clicked"
            # "2"
            # "1"
            # "Descr."
            # "Descr."
            # "VMON1  x4 \nVMON2  x2\nIMON1    x4\nIMON2    x2"
            # "Needle gauge Voltage displays"
            # "1"
            # "2"
            # "1"
            # "2"
            # "Reads new V and A every N cycles,\nor passes previous values"
            # "High Voltage"
            n92 = Unbundle(w363) -> ("VISA resource name out"=w338:refnum<visa-resource-name>, "error out"=w362:errorcluster)
            n93 = Unbundle(w360) -> ("VISA resource name out"=w337:refnum<visa-resource-name>, "error out"=w359:errorcluster)
            n94 = Quotient & Remainder(x=w356, y="Read V every N cycles") -> (x-y*floor(x/y)=w322:i32)  [unwired: 1 out]
            n95 = Build Array (concatenate)("VSet (V)", "VMax (V)", "IMax (uA)") -> (w327:dbl[])
            n96 = case shown="0" w322 {
              tunnel: w338 -> [w472 _]
              tunnel: w362 -> [w471 w480]
              tunnel: w361 -> [_ w476]
              tunnel: w337 -> [w462 _]
              tunnel: w359 -> [w460 w481]
              tunnel: [w459 w481] -> w339
              tunnel: [w468 w480] -> w340
              tunnel: [w467 w476] -> w342
              tunnel: [w465 w477] -> w358
              tunnel: [w463 w473] -> w357
              frame 0 {
                # "All data x12"
                # "Voltages x6"
                # "Currents x6"
                # "Read"
                n97 = call "READ_SUPPLY.vi"("VISA resource name"=w472, "Board address"=u8 0, "NChannels"=u8 4, "error in (no error)"=w471) -> ("VMon values (V)"=w466:dbl[], "IMon values (uA)"=w464:dbl[], "error out"=w468:errorcluster)  [unwired: 9 in]
                n98 = call "Read_CAEN_ch1_and_2.vi"("VISA resource name in"=w462, "Board address"=u8 0, "error in"=w460) -> ("VMon values (V)"=w458:dbl[], "IMon values (uA)"=w457:dbl[], "error out"=w459:errorcluster)  [unwired: 4 in, 1 out]
                n99 = Build Array (concatenate)(w464, w457) -> (w463:dbl[])
                n100 = Build Array (concatenate)(w466, w458) -> (w465:dbl[])
                n101 = Build Array (concatenate)(w466, w458, w464, w457) -> (w467:dbl[])
              }
              frame 1, Default {
                # "Don't read: pass previous"
                n102 = Array Subset(array=w476, index=0, length=6) -> (w477:dbl[])
                n103 = Array Subset(array=w476, index=6, length=6) -> (w473:dbl[])
              }
            }
            "Voltages" <- w358
            "Vmon (V)" <- w358
            "IMon (uA)" <- w357
            n104 = Build Array("Apply Voltage", "Set to zero", "Kill voltage") -> (w321:bool[])
            n105 = Search 1D Array(1D array=w321, element=TRUE) -> (index of element=w341:i32)  [unwired: 1 in]
            n106 = case shown="0" w341 {
              tunnel: w340 -> [w381 w411 w441 w453]
              tunnel: w339 -> [w367 w400 w430 w455]
              tunnel: w338 -> [w377 w408 w438 w456]
              tunnel: w337 -> [w365 w398 w428 w454]
              tunnel: [w378 w409 w439 w453] -> w331
              tunnel: [w377 w408 w438 w456] -> w336
              tunnel: [w364 w397 w427 w455] -> w333
              tunnel: [w365 w398 w428 w454] -> w334
              tunnel: "VSet (V)" -> [w375 _ w436 _]
              tunnel: "VMax (V)" -> [w374 w406 _ _]
              tunnel: "IMax (uA)" -> [w373 w405 w435 _]
              frame 0 {
                w366 = 4 ("length")
                w371 = 2 ("length")
                w372 = 4 ("length")
                # "CAEN 2: Top gate, Bottom gate"
                # "CAEN 1 set values:\nPMT1&2, Anode, Cathode"
                # "Apply voltage"
                n107 = Array Subset(array=w375, length=w372) -> (w380:dbl[])  [unwired: 1 in]
                n108 = Array Subset(array=w374, length=w372) -> (w379:dbl[])  [unwired: 1 in]
                n109 = Array Subset(array=w373, length=w372) -> (w376:dbl[])  [unwired: 1 in]
                n110 = Array Subset(array=w373, index=w366, length=w371) -> (w368:dbl[])
                n111 = Array Subset(array=w375, index=w366, length=w371) -> (w370:dbl[])
                n112 = Array Subset(array=w374, index=w366, length=w371) -> (w369:dbl[])
                n113 = for {
                  tunnel: w377 -> [w391]
                  tunnel: w381 -> [w390]
                  tunnel: w380 -> [w387] mode=indexing
                  tunnel: w379 -> [w385] mode=indexing
                  tunnel: w376 -> [w384] mode=indexing
                  tunnel: [w383] -> w378
                  i -> [w392]
                  n114 = call "SET_SUPPLY_CHANNEL.vi"("VISA resource name"=w391, "Voltage Level (0.0 V)"=w387, "Enable (OFF)"=TRUE, "Board address"=u8 0, "NChannels"=u8 4, "Channel (0)"=w392, "error in (no error)"=w390, "Voltage Max (0.0 V)"=w385, "Current Limit (0.00 uA)"=w384) -> ("error out"=w383:errorcluster)  [unwired: 6 in]
                }
                n115 = for {
                  tunnel: w365 -> [_]
                  tunnel: w367 -> [w382]
                  tunnel: w370 -> [_] mode=indexing
                  tunnel: w369 -> [_] mode=indexing
                  tunnel: w368 -> [_] mode=indexing
                  tunnel: [w382] -> w364
                  # "CAEN 2 SET SUPPLY"
                }
              }
              frame 1 {
                w393 = 0 ("length")
                w395 = 0 ("length")
                w399 = 4 ("length")
                w403 = 2 ("length")
                w404 = 4 ("length")
                # "CAEN 2: Top gate, Bottom gate"
                # "CAEN 1 values:\nPMT1&2, Anode, Cathode"
                # "Set V to zero"
                n116 = Build Array(w395, w395, w395, w395) -> (w396:i32[])
                n117 = Array Subset(array=w405, length=w404) -> (w407:dbl[])  [unwired: 1 in]
                n118 = Array Subset(array=w406, length=w404) -> (w410:dbl[])  [unwired: 1 in]
                n119 = Build Array(w393, w393) -> (w394:i32[])
                n120 = Array Subset(array=w405, index=w399, length=w403) -> (w401:dbl[])
                n121 = Array Subset(array=w406, index=w399, length=w403) -> (w402:dbl[])
                n122 = for {
                  tunnel: w408 -> [w421]
                  tunnel: w411 -> [w420]
                  tunnel: w396 -> [w417] mode=indexing
                  tunnel: w410 -> [w415] mode=indexing
                  tunnel: w407 -> [w414] mode=indexing
                  tunnel: [w413] -> w409
                  i -> [w422]
                  n123 = call "SET_SUPPLY_CHANNEL.vi"("VISA resource name"=w421, "Voltage Level (0.0 V)"=w417, "Enable (OFF)"=TRUE, "Board address"=u8 0, "NChannels"=u8 4, "Channel (0)"=w422, "error in (no error)"=w420, "Voltage Max (0.0 V)"=w415, "Current Limit (0.00 uA)"=w414) -> ("error out"=w413:errorcluster)  [unwired: 6 in]
                }
                n124 = for {
                  tunnel: w398 -> [_]
                  tunnel: w400 -> [w412]
                  tunnel: w394 -> [_] mode=indexing
                  tunnel: w402 -> [_] mode=indexing
                  tunnel: w401 -> [_] mode=indexing
                  tunnel: [w412] -> w397
                  # "CAEN 2 SET SUPPLY CH 2"
                }
              }
              frame 2 {
                w424 = 0 ("length")
                w426 = 0 ("length")
                w429 = 4 ("length")
                w433 = 2 ("length")
                w434 = 4 ("length")
                # "CAEN 2: Top gate, Bottom gate"
                # "CAEN 1 values:\nPMT1&2, Anode, Cathode"
                # "Set VMax to zero, \"Kill\""
                n125 = Array Subset(array=w435, length=w434) -> (w437:dbl[])  [unwired: 1 in]
                n126 = Array Subset(array=w436, length=w434) -> (w440:dbl[])  [unwired: 1 in]
                n127 = Build Array(w426, w426, w426, w426) -> (w425:i32[])
                n128 = Array Subset(array=w435, index=w429, length=w433) -> (w431:dbl[])
                n129 = Array Subset(array=w436, index=w429, length=w433) -> (w432:dbl[])
                n130 = Build Array(w424, w424) -> (w423:i32[])
                n131 = for {
                  tunnel: w438 -> [w451]
                  tunnel: w441 -> [w450]
                  tunnel: w440 -> [w447] mode=indexing
                  tunnel: w425 -> [w445] mode=indexing
                  tunnel: w437 -> [w444] mode=indexing
                  tunnel: [w443] -> w439
                  i -> [w452]
                  n132 = call "SET_SUPPLY_CHANNEL.vi"("VISA resource name"=w451, "Voltage Level (0.0 V)"=w447, "Enable (OFF)"=TRUE, "Board address"=u8 0, "NChannels"=u8 4, "Channel (0)"=w452, "error in (no error)"=w450, "Voltage Max (0.0 V)"=w445, "Current Limit (0.00 uA)"=w444) -> ("error out"=w443:errorcluster)  [unwired: 6 in]
                }
                n133 = for {
                  tunnel: w428 -> [_]
                  tunnel: w430 -> [w442]
                  tunnel: w432 -> [_] mode=indexing
                  tunnel: w423 -> [_] mode=indexing
                  tunnel: w431 -> [_] mode=indexing
                  tunnel: [w442] -> w427
                  # "CAEN 2 SET SUPPLY CH 2"
                }
              }
              frame 3, Default {
                # "\"Executes\" if none of the three buttons have been clicked"
                # "Do nothing"
              }
            }
            n134 = Index Array(array=w342, index #1=0 ("index"), index #2=1 ("index"), index #3=2 ("index"), index #4=3 ("index"), index #5=4 ("index"), index #6=5 ("index")) -> (element #1=→"PMT 1":dbl, element #2=→"PMT 2":dbl, element #3=→"Anode":dbl, element #4=→"Cathode":dbl, element #5=→"Top gate":dbl, element #6=→"Bottom gate":dbl)
            n135 = Bundle("VISA resource name out"=w336, "error out"=w331) -> (w335:T5)  [unwired: 1 in]
            n136 = Bundle("VISA resource name out"=w334, "error out"=w333) -> (w332:T5)  [unwired: 1 in]
          }
          frame #4 {
            # "Descr."
            # "Reset anode"
            n137 = Search 1D Array(1D array=w492, element=TRUE) -> (index of element=w483:i32)  [unwired: 1 in]
            n138 = Not Equal?(x=w483, y=-1) -> (x != y?=w488:bool)
            n139 = case shown="True" "Reset anode" {
              tunnel: w491 -> [_ w515]
              tunnel: w490 -> [_ w527]
              tunnel: w489 -> [_ w496]
              tunnel: w488 -> [_ w517]
              tunnel: [w493 w497] -> w485
              frame False {
                # "Anode Reset Routine inactive:\nkeep timers up to date so activating\nroutine will correctly initiate the timers."
                n140 = Get Date/Time In Seconds() -> (seconds since 1Jan1904=w495:timestamp)
                n141 = To Double Precision Float(number=w495) -> (double precision float=w494:dbl)
                n142 = Build Array(w494, w494) -> (w493:dbl[])
              }
              frame True {
                # "0: 1st timer reset, 1: both timers reset, else: do nothing"
                # "Timers"
                # "0: Set to zero, 1: set to value, else: do nothing"
                # "Resetting the timers"
                # "Change Anode Voltage"
                # "Anode Imax"
                # "Anode Vmax"
                # "Anode Vset"
                # "Current time > total routine time?"
                # "Current time > target autokill time?"
                n143 = Get Date/Time In Seconds() -> (seconds since 1Jan1904=w529:timestamp)
                n144 = Index Array(array=w515, index #1=0 ("index"), index #2=1 ("index")) -> (element #1=w509:dbl, element #2=w511:dbl)
                n145 = To Double Precision Float(number=w529) -> (double precision float=w510:dbl)
                n146 = Multiply(x="Kill every Y minutes", y=60) -> (x*y=w507:i32)
                n147 = Unbundle(w527) -> ("VISA resource name out"=w526:refnum<visa-resource-name>, "error out"=w525:errorcluster)
                n148 = Subtract(x=w510, y=w509) -> (x-y=w508:dbl)
                n149 = Subtract(x=w510, y=w511) -> (x-y=w499:dbl)
                n150 = Add(x=w507, y="Keep off for X seconds") -> (x+y=w498:i32)
                n151 = Greater?(x=w508, y=w507) -> (0:w501:bool)
                "Killed" <- w501
                n152 = Greater?(x=w499, y=w498) -> (0:w502:bool)
                "Restarted" <- w502
                n153 = Or(x=w502, y=w517) -> (x .or. y?=w505:bool)
                n154 = Build Array(w501, w502) -> (w519:bool[])
                n155 = Build Array(w501, w505) -> (w506:bool[])
                n156 = Index Array(array=w496, index #1=2 ("index"), index #2=8 ("index"), index #3=14 ("index")) -> (element #1=w522:dbl, element #2=w520:dbl, element #3=w521:dbl)
                n157 = Search 1D Array(1D array=w519, element=TRUE) -> (index of element=w518:i32)  [unwired: 1 in]
                n158 = Search 1D Array(1D array=w506, element=TRUE) -> (index of element=w503:i32)  [unwired: 1 in]
                n159 = case shown="0" w518 {
                  tunnel: w522 -> [_ w554 _]
                  tunnel: w520 -> [w542 w553 _]
                  tunnel: w521 -> [w544 w552 _]
                  tunnel: w526 -> [w550 w557 _]
                  tunnel: w525 -> [w549 w556 _]
                  frame 0 {
                    # "Anode Vset to zero"
                    n160 = call "SET_SUPPLY_CHANNEL.vi"("VISA resource name"=w550, "Voltage Level (0.0 V)"=0.0, "Enable (OFF)"=TRUE, "Board address"=u8 0, "NChannels"=u8 4, "Channel (0)"=u8 2, "error in (no error)"=w549, "Voltage Max (0.0 V)"=w542, "Current Limit (0.00 uA)"=w544) -> ("error out"=w543:errorcluster)  [unwired: 6 in]
                    n161 = call <vilib>:"Simple Error Handler.vi"("error in (no error)"=w543) -> ()  [unwired: 4 in, 5 out]
                  }
                  frame 1 {
                    # "Anode Vset applied"
                    n162 = call "SET_SUPPLY_CHANNEL.vi"("VISA resource name"=w557, "Voltage Level (0.0 V)"=w554, "Enable (OFF)"=TRUE, "Board address"=u8 0, "NChannels"=u8 4, "Channel (0)"=u8 2, "error in (no error)"=w556, "Voltage Max (0.0 V)"=w553, "Current Limit (0.00 uA)"=w552) -> ("error out"=w551:errorcluster)  [unwired: 6 in]
                    n163 = call <vilib>:"Simple Error Handler.vi"("error in (no error)"=w551) -> ()  [unwired: 4 in, 5 out]
                  }
                  frame 2, Default {
                    # "Do nothing"
                  }
                }
                n164 = case shown="0" w503 {
                  tunnel: [w531 w537 w540] -> w497
                  tunnel: w515 -> [w535 _ w540]
                  frame 0 {
                    # "Only reset 1st timer, so it\ndoesn't stay True and lock-\nout 2nd check"
                    n165 = Get Date/Time In Seconds() -> (seconds since 1Jan1904=w534:timestamp)
                    n166 = Index Array(array=w535, index=1) -> (element=w532:dbl)
                    n167 = To Double Precision Float(number=w534) -> (double precision float=w533:dbl)
                    n168 = Build Array(w533, w532) -> (w531:dbl[])
                  }
                  frame 1 {
                    # "Reset timers if any button is pressed,\nor if the anode ramps up again"
                    n169 = Get Date/Time In Seconds() -> (seconds since 1Jan1904=w539:timestamp)
                    n170 = To Double Precision Float(number=w539) -> (double precision float=w538:dbl)
                    n171 = Build Array(w538, w538) -> (w537:dbl[])
                  }
                  frame 2, Default {
                    # "Time difference grows \nlarger for now"
                  }
                }
              }
            }
            "Anode times" <- w485
            n172 = To Time Stamp(1:w485) -> (0:→"Anode times 2":timestamp[])
            "?" <- "Reset anode"
          }
          frame #5 {
            # "Descr."
            # "Moving averages"
            # "Plots heater power vs. t"
            # "Historic graphs: Phase, Pressure, Flow, Heater, Temperature"
            # "Plots flow vs. t"
            # "Plots three pressures vs. t in one graph"
            # "Non-historic Temperature + Det. Pressure"
            # "Det., Low, High, Flow, Heater\nentire columns"
            # "Latest readings (NI, LS)"
            # "Single Temp.'s"
            # "Single Temp.'s"
            # "Updated TOBA"
            # "Descr."
            # "Latest Detector Pressure"
            # "Plots individual lists of Temp. vs. t"
            # "Plots and moving averages"
            n173 = Build Array (concatenate)(w604, w597) -> (w562:dbl[][])
            "TOBA appended" <- w562
            n174 = case shown="\"Average 15 to 20\", Default" "Temp. Channel selector" {
              tunnel: w597 -> [w667 w669 w672 w675 w678 w681 w684 w687 w694]
              tunnel: [w665 w668 w671 w674 w677 w680 w683 w686 w689] -> w607
              frame "Channel 15" {
                n175 = Index Array(array=w667, index=14) -> (element=w665:dbl)
              }
              frame "Channel 16" {
                n176 = Index Array(array=w669, index=15) -> (element=w668:dbl)
              }
              frame "Channel 17" {
                n177 = Index Array(array=w672, index=16) -> (element=w671:dbl)
              }
              frame "Channel 18" {
                n178 = Index Array(array=w675, index=17) -> (element=w674:dbl)
              }
              frame "Channel 19" {
                n179 = Index Array(array=w678, index=18) -> (element=w677:dbl)
              }
              frame "Channel 20" {
                n180 = Index Array(array=w681, index=19) -> (element=w680:dbl)
              }
              frame "Channel A" {
                n181 = Index Array(array=w684, index=20) -> (element=w683:dbl)
              }
              frame "Channel B" {
                n182 = Index Array(array=w687, index=21) -> (element=w686:dbl)
              }
              frame "Average 15 to 20", Default {
                w690 = 6 ("length")
                n183 = Array Subset(array=w694, index=14, length=w690) -> (w692:dbl[])
                n184 = Add Array Elements(numeric array=w692) -> (sum=w691:dbl)
                n185 = Divide(x=w691, y=w690) -> (x/y=w689:dbl)
              }
            }
            n186 = case shown="\"Channel 17\", Default" "Temperature Channel selector" {
              tunnel: w562 -> [w612 w615 w618 w621 w624 w627 w630 w633]
              tunnel: [w611 w614 w617 w620 w623 w626 w629 w632] -> w594
              frame "Channel 15" {
                n187 = Index Array(array=w612, index (col)=14) -> (element=w611:dbl[])  [unwired: 1 in]
              }
              frame "Channel 16" {
                n188 = Index Array(array=w615, index (col)=15) -> (element=w614:dbl[])  [unwired: 1 in]
              }
              frame "Channel 17", Default {
                n189 = Index Array(array=w618, index (col)=16) -> (element=w617:dbl[])  [unwired: 1 in]
              }
              frame "Channel 18" {
                n190 = Index Array(array=w621, index (col)=17) -> (element=w620:dbl[])  [unwired: 1 in]
              }
              frame "Channel 19" {
                n191 = Index Array(array=w624, index (col)=18) -> (element=w623:dbl[])  [unwired: 1 in]
              }
              frame "Channel 20" {
                n192 = Index Array(array=w627, index (col)=19) -> (element=w626:dbl[])  [unwired: 1 in]
              }
              frame "Channel A" {
                n193 = Index Array(array=w630, index (col)=20) -> (element=w629:dbl[])  [unwired: 1 in]
              }
              frame "Channel B" {
                n194 = Index Array(array=w633, index (col)=21) -> (element=w632:dbl[])  [unwired: 1 in]
              }
            }
            n195 = for {
              N: 22 -> [_]
              tunnel: w577 -> [w699]
              tunnel: [w698] -> w609 mode=indexing
              tunnel: w562 -> [w697]
              i -> [w696]
              n196 = Index Array(array=w697, index (col)=w696) -> (element=w695:dbl[])  [unwired: 1 in]
              n197 = Bundle(w699, w695) -> (w698:cluster{timestamp[], dbl[]})  [unwired: 1 in]
            }
            "Temperature" <- w609
            n198 = Index Array(array=w562, index (col) #1=23 ("disabled index (col)"), index (col) #2=24 ("index (col)"), index (col) #3=25 ("index (col)"), index (col) #4=26 ("index (col)"), index (col) #5=22 ("index (col)")) -> (element #1=w576:dbl[], element #2=w589:dbl[], element #3=w588:dbl[], element #4=w569:dbl[], element #5=w579:dbl[])  [unwired: 5 in]
            n199 = Index Array(array=w597, index=23) -> (element=w598:dbl)
            n200 = Bundle(w594, w576) -> (w593:cluster{dbl[], dbl[]})  [unwired: 1 in]
            n201 = Bundle("Waveform"=w607, "Waveform"=w598) -> (w606:cluster{"Waveform":dbl, "Waveform":dbl})  [unwired: 1 in]
            n202 = Bundle(w577, w576) -> (w587:cluster{timestamp[], dbl[]})  [unwired: 1 in]
            n203 = Bundle(w577, w589) -> (w586:cluster{timestamp[], dbl[]})  [unwired: 1 in]
            n204 = Bundle(w577, w588) -> (w585:cluster{timestamp[], dbl[]})  [unwired: 1 in]
            n205 = Bundle(w577, w569) -> (w582:cluster{timestamp[], dbl[]})  [unwired: 1 in]
            n206 = Bundle(w577, w579) -> (w578:cluster{timestamp[], dbl[]})  [unwired: 1 in]
            n207 = Build Array(w606) -> (→"Phase Diagram":cluster{"Waveform":dbl, "Waveform":dbl}[])
            n208 = Build Array(w593) -> (→"Historical Large Phase Diagram":cluster{dbl[], dbl[]}[])
            n209 = Build Array(w587, w586, w585) -> (→"Pressure":cluster{timestamp[], dbl[]}[])
            n210 = Build Array(w582) -> (→"Flow (SLPM)":cluster{timestamp[], dbl[]}[])
            n211 = Build Array(w578) -> (→"Heater power (%)":cluster{timestamp[], dbl[]}[])
            n212 = case shown="\"Average 15 to 20\", Default" "Temperature Channel selector" {
              tunnel: w597 -> [w637 w639 w642 w645 w648 w651 w654 w657 w664]
              tunnel: [w635 w638 w641 w644 w647 w650 w653 w656 w659] -> w602
              frame "Channel 15" {
                n213 = Index Array(array=w637, index=14) -> (element=w635:dbl)
              }
              frame "Channel 16" {
                n214 = Index Array(array=w639, index=15) -> (element=w638:dbl)
              }
              frame "Channel 17" {
                n215 = Index Array(array=w642, index=16) -> (element=w641:dbl)
              }
              frame "Channel 18" {
                n216 = Index Array(array=w645, index=17) -> (element=w644:dbl)
              }
              frame "Channel 19" {
                n217 = Index Array(array=w648, index=18) -> (element=w647:dbl)
              }
              frame "Channel 20" {
                n218 = Index Array(array=w651, index=19) -> (element=w650:dbl)
              }
              frame "Channel A" {
                n219 = Index Array(array=w654, index=20) -> (element=w653:dbl)
              }
              frame "Channel B" {
                n220 = Index Array(array=w657, index=21) -> (element=w656:dbl)
              }
              frame "Average 15 to 20", Default {
                w660 = 6 ("length")
                n221 = Array Subset(array=w664, index=14, length=w660) -> (w662:dbl[])
                n222 = Add Array Elements(numeric array=w662) -> (sum=w661:dbl)
                n223 = Divide(x=w661, y=w660) -> (x/y=w659:dbl)
              }
            }
            n224 = Reverse 1D Array(array=w576) -> (reversed array=w575:dbl[])
            n225 = Reverse 1D Array(array=w569) -> (reversed array=w571:dbl[])
            n226 = Array Subset(array=w575, length="N samples") -> (w564:dbl[])  [unwired: 1 in]
            n227 = Array Subset(array=w571, length="N samples") -> (w566:dbl[])  [unwired: 1 in]
            n228 = Array Size(array=w566) -> (size(s)=w565:i32)
            n229 = Array Size(array=w564) -> (size(s)=w563:i32)
            n230 = Add Array Elements(numeric array=w566) -> (sum=w570:dbl)
            n231 = Add Array Elements(numeric array=w564) -> (sum=w574:dbl)
            n232 = Bundle("Waveform"=w602, "Waveform"=w598) -> (w603:cluster{"Waveform":dbl, "Waveform":dbl})  [unwired: 1 in]
            n233 = Divide(x=w570, y=w565) -> (x/y=→"Average Flow (SLPM)":dbl)
            n234 = Divide(x=w574, y=w563) -> (x/y=→"Moving average Det. P":dbl)
            n235 = Build Array(w603) -> (→"Large Phase Diagram":cluster{"Waveform":dbl, "Waveform":dbl}[])
          }
          frame #6 {
            # "------------OBSOLETE------------\nTemperatures (20),      NI Box;\nTemperatures (4),  Lakeshore;\nHeater Power,       Lakeshore;\nPressures (4),               NI Box;\nSetpoint,               Lakeshore;\nCurrent time (s)               ---   ;\nCycle time (s)                   ---   ;"
            # "Saving data"
            n236 = Get Date/Time In Seconds() -> (seconds since 1Jan1904=w713:timestamp)
            n237 = To Double Precision Float(number=w713) -> (double precision float=w712:dbl)
            n238 = Build Array (concatenate)(w715, w714, w712, w711, w710) -> (w709:dbl[])
            n239 = Get Date/Time String() -> (date string=w703:string)  [unwired: 3 in, 1 out]
            n240 = Build Path(base path=path "D:/Log_data/SC_LOG", name or relative path=w703) -> (appended path=w702:path)
            n241 = Format Date/Time String() -> (date/time string=w707:string)  [unwired: 3 in]
            n242 = Array To Spreadsheet String(array=w709, 3:"%.3f" ("format string")) -> (spreadsheet string=w705:string)  [unwired: 1 in]
            n243 = Concatenate Strings(w707, "\t", w705) -> (w701:string)
            n244 = call <vilib>:"Write Spreadsheet String.vi"("append to file? (new file:F)"=TRUE, "spreadsheet string"=w701, "file path (dialog if empty)"=w702) -> ()  [unwired: 7 in, 2 out]
          }
          frame #7 {
            # "Alarm conditions (Temp)"
            # "NI mod2 & 3 status go here"
            # "Check alarms and UPS"
            n245 = Unbundle By Name(w744) -> ("error out.status"=w741:bool)
            "LakeShore status" <- w741
            n246 = Unbundle By Name(w746) -> ("error out.status"=w740:bool)
            "CAEN 1 status" <- w740
            n247 = Unbundle By Name(w745) -> ("error out.status"=w739:bool)
            "CAEN 2 status" <- w739
            n248 = Unbundle By Name(w742) -> ("error out.status"=w738:bool)
            "NI mod1 (P) status" <- w738
            n249 = Index Array(array=w727, index=23) -> (element=w733:dbl)
            n250 = Build Array(w741, w740, w739, w738) -> (w737:bool[])
            n251 = Or Array Elements(Boolean array=w737) -> (logical OR=→"Comm. status":bool)
            n252 = Greater?(x=w733, y="Overpressure threshold") -> (0:w731:bool)
            n253 = Less?(x=w733, y="Underpressure threshold") -> (x < y?=w730:bool)
            n254 = Or(x=w731, y=w730) -> (x .or. y?=w729:bool)
            n255 = And(x="Detector P", y=w729) -> ()  [unwired: 1 out]
            n256 = Array Subset(array=w727, index=14, length=6) -> (w724:dbl[])
            n257 = Build Array("T 15", "T 16", "T 17", "T 18", "T 19", "T 20") -> (w716:bool[])
            n258 = for {
              tunnel: w724 -> [w751] mode=indexing
              tunnel: [w748] -> w723 mode=indexing
              tunnel: w716 -> [w747] mode=indexing
              n259 = Greater?(x=w751, y="High Temp threshold") -> (0:w750:bool)
              n260 = Less?(x=w751, y="Low Temp threshold") -> (x < y?=w749:bool)
              n261 = Or(x=w750, y=w749) -> (x .or. y?=w748:bool)
              n262 = And(x=w747, y=w748) -> ()  [unwired: 1 out]
            }
            n263 = Index Array(array=w723) -> ()  [unwired: 1 in, 1 out]
          }
        }
        n264 = Decrement(x="Cycles to execute") -> (x-1=w163:dbl)
        n265 = Greater?(x=w175, y=w163) -> (0:w150:bool)
        n266 = Or(x=w150, y="stop") -> (x .or. y?=w178:bool)
      }
      "TOBA tester" <- w140
    }
    frame True {
    }
  }
  n267 = Array Size(array=w21) -> (size(s)=w24:i32)
  n268 = Decrement(x=w24) -> (x-1=w23:i32)
  n269 = flat-sequence {
    tunnel: w10 -> [w782]
    tunnel: w6 -> [w773]
    tunnel: w5 -> [w770]
    tunnel: w4 -> [w765]
    frame #0 {
      w778 = u16 2 items=["1"=1, "2"=2] ("Heater Output (1:1)")
      w779 = u16 0 items=["Off", "Low (On)", "Medium", "High"] ("Range (0:Off)")
      # "Turn off heater, shutdown COM"
      # "Error Handling and Post-Processing (EHaPP)"
      n270 = Unbundle(w782) -> ("VISA resource name out"=w781:refnum<visa-resource-name>, "error out"=w780:errorcluster)
      n271 = Unbundle(w773) -> ("VISA resource name out"=w772:refnum<visa-resource-name>, "error out"=w771:errorcluster)
      n272 = Unbundle(w770) -> ("VISA resource name out"=w769:refnum<visa-resource-name>, "error out"=w768:errorcluster)
      n273 = Unbundle(w765) -> ("task out"=w763:refnum<k21>, "error out"=w762:errorcluster)
      n274 = call <vilib>:"DAQmx Stop Task.vi"("task/channels in"=w763, "error in"=w762) -> ("task out"=w761:refnum<k21>, "error out"=w760:errorcluster)  [unwired: 12 in]
      n275 = call <instrlib>:"Configure Output Range and Manual Value.vi"("VISA resource name"=w781, "Heater Output (1:1)"=w778, "Range (0:Off)"=w779, "Manual Output (0.00 %)"=0.0, "error in (no error)"=w780) -> ("VISA resource name out"=w776:refnum<visa-resource-name>, "error out"=w775:errorcluster)  [unwired: 9 in]
      n276 = call <instrlib>:"Close.vi"("error in (no error)"=w771, "VISA resource name"=w772) -> ("error out"=w767:errorcluster)  [unwired: 9 in]
      n277 = call <instrlib>:"Close.vi"("error in (no error)"=w768, "VISA resource name"=w769) -> ("error out"=w766:errorcluster)  [unwired: 9 in]
      n278 = call <vilib>:"DAQmx Clear Task.vi"("task in"=w761, "error in"=w760) -> ("error out"=w764:errorcluster)  [unwired: 13 in]
      n279 = call <instrlib>:"Close.vi"("error in (no error)"=w775, "VISA resource name"=w776) -> ("error out"=w774:errorcluster)  [unwired: 9 in]
      n280 = call <vilib>:"Simple Error Handler.vi"("error in (no error)"=w774) -> ()  [unwired: 4 in, 5 out]
      n281 = call <vilib>:"Simple Error Handler.vi"("error in (no error)"=w767) -> ()  [unwired: 4 in, 5 out]
      n282 = call <vilib>:"Simple Error Handler.vi"("error in (no error)"=w766) -> ()  [unwired: 4 in, 5 out]
      n283 = call <vilib>:"Simple Error Handler.vi"("error in (no error)"=w764) -> ()  [unwired: 4 in, 5 out]
    }
  }
  n284 = Index Array(array=w21, index #1=w23, index #2=1 ("index")) -> (element #1=w22:timestamp, element #2=w2:timestamp)
  n285 = To Double Precision Float(number=w22) -> (double precision float=w20:dbl)
  n286 = To Double Precision Float(number=w2) -> (double precision float=w19:dbl)
  n287 = Subtract(x=w20, y=w19) -> ()  [unwired: 1 out]
  "Started up?" <- w15
